vi "MetaServerTCPGo.vi"(8 "error in (no error)":errorcluster, 10 "runs":i32=3, 11 "steps":i32=10) -> (0 "error out":errorcluster)   [LabVIEW 2017]
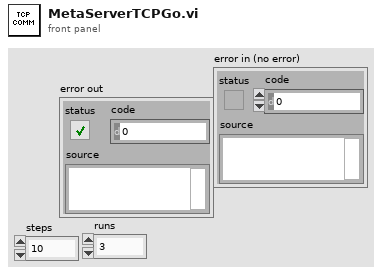
[diagram p1: front panel]
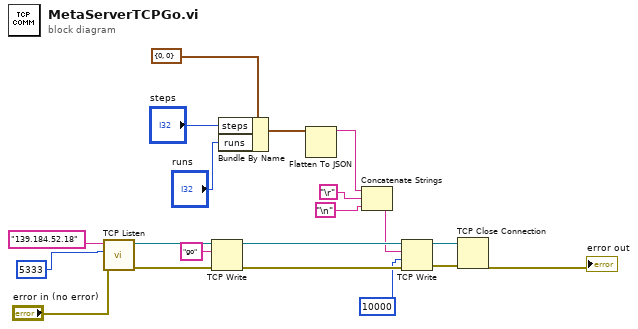
[diagram p0: block diagram]
diagram:
  n1 = call <vilib>:"TCP Listen.vi"("error in (no error)"="error in (no error)", "port"=u16 5333 ("remote port or service name"), "service name"="139.184.52.18" ("address")) -> ("error out"=w17:errorcluster, "connection ID"=w16:refnum<k5>)  [unwired: 4 in, 3 out]
  n2 = TCP Write(connection ID=w16, data in="go", error in (no error)=w17) -> (connection ID out=w19:refnum<k5>, error out=w18:errorcluster)  [unwired: 1 in, 1 out]
  n3 = Bundle By Name(cluster=cluster{"steps":i32, "runs":i32} {"steps"=0, "runs"=0}, "steps"="steps", "runs"="runs") -> (w3:cluster{"steps":i32, "runs":i32})
  n4 = Flatten To JSON(anything=w3) -> (JSON string=w10:string)  [unwired: 2 in, 1 out]
  n5 = Concatenate Strings(w10, "\r", "\n") -> (w9:string)
  n6 = TCP Write(connection ID=w19, data in=w9, error in (no error)=w18, 9:10000 ("timeout ms (25000)")) -> (connection ID out=w14:refnum<k5>, error out=w13:errorcluster)  [unwired: 1 out]
  n7 = TCP Close Connection(connection ID=w14, error in (no error)=w13) -> (error out=→"error out":errorcluster)  [unwired: 1 in, 1 out]
